vi "Hardware - NI 9755-1 (NOx) Host.vi"() -> ()   [LabVIEW 2015, in "ECS-Host.lvlib"]
uses:
  ECS-Host.lvlib
panel:
  out "RxIDActual":u32 format="%.0x"
  out "FPGAInterfaceError":bool
  in  "Sensor2RxID":u32 format="%.0x"
  out "Sensor2HeaterModeStatus":T1(ring)
  out "Sensor2O2CircuitStatus":enum32{"OPEN WIRE", "SHORT CIRCUIT", "NO ERROR"}(ring)
  out "Sensor2NOxCircuitStatus":enum32{"OPEN WIRE", "SHORT CIRCUIT", "NO ERROR"}(ring)
  out "Sensor2HeaterCircuitStatus":enum32{"OPEN WIRE", "SHORT CIRCUIT", "NO ERROR"}(ring)
  out "Sensor2O2SignalStatus":T2(ring)
  out "Sensor2NOxSignalStatus":T2(ring)
  out "Sensor2TemperatureStatus":T3(ring)
  out "Sensor2O2":sgl caption="[%]"
  out "Sensor2NOx":i32 caption="[ppm]"
  out "Sensor2SupplyStatus":T4(ring)
  in  "Sensor2_E":bool
  out "Sensor2Present":bool
  in  "TxID":u32 format="%.0x"
  in  "Sensor1RxID":u32 format="%.0x"
  out "Sensor1HeaterModeStatus":T1(ring)
  out "Sensor1O2CircuitStatus":enum32{"OPEN WIRE", "SHORT CIRCUIT", "NO ERROR"}(ring)
  out "Sensor1NOxCircuitStatus":enum32{"OPEN WIRE", "SHORT CIRCUIT", "NO ERROR"}(ring)
  out "Sensor1HeaterCircuitStatus":enum32{"OPEN WIRE", "SHORT CIRCUIT", "NO ERROR"}(ring)
  out "Sensor1O2SignalStatus":T2(ring)
  out "Sensor1NOxSignalStatus":T2(ring)
  out "Sensor1TemperatureStatus":T3(ring)
  out "Sensor1O2":sgl caption="[%]"
  out "Sensor1NOx":i32 caption="[ppm]"
  out "Sensor1SupplyStatus":T4(ring)
  in  "Sensor1_E":bool
  out "Sensor1Present":bool
  in  "CAN0_Restart":bool
  # "NOx1"
  # "NOx2"
  # "Rx ID"
  # "Rx ID"
  # "Supply"
  # "Supply"
  # "Temperature"
  # "Temperature"
  # "NOx Signal"
  # "NOx Signal"
  # "O2 Signal"
  # "O2 Signal"
  # "Heater Mode"
  # "Heater Mode"
  # "Heater Circuit"
  # "Heater Circuit"
  # "NOx Circuit"
  # "NOx Circuit"
  # "O2 Circuit"
  # "O2 Circuit"
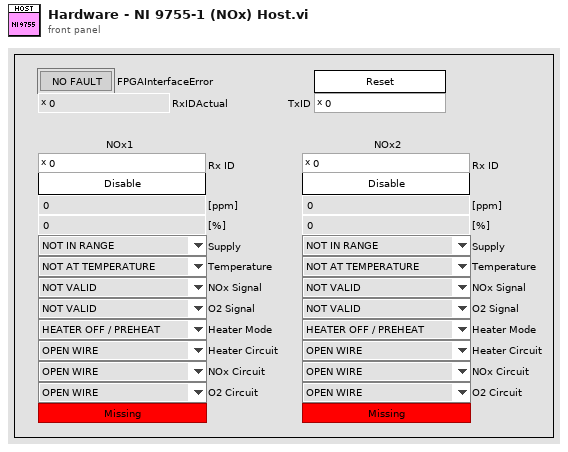
[diagram p1: front panel]
types:
  T1 = enum32{"HEATER OFF / PREHEAT", "HEATER SLOPE 1 OR 2", "HEATER SLOPE 3 OR 4", "AUTO MODE"}
  T2 = enum32{"NOT VALID", "VALID", "ERROR", "NOT AVAILABLE"}
  T3 = enum32{"NOT AT TEMPERATURE", "AT TEMPERATURE", "ERROR", "NOT AVAILABLE"}
  T4 = enum32{"NOT IN RANGE", "SUPPLY IN RANGE", "ERROR", "NOT AVAILABLE"}
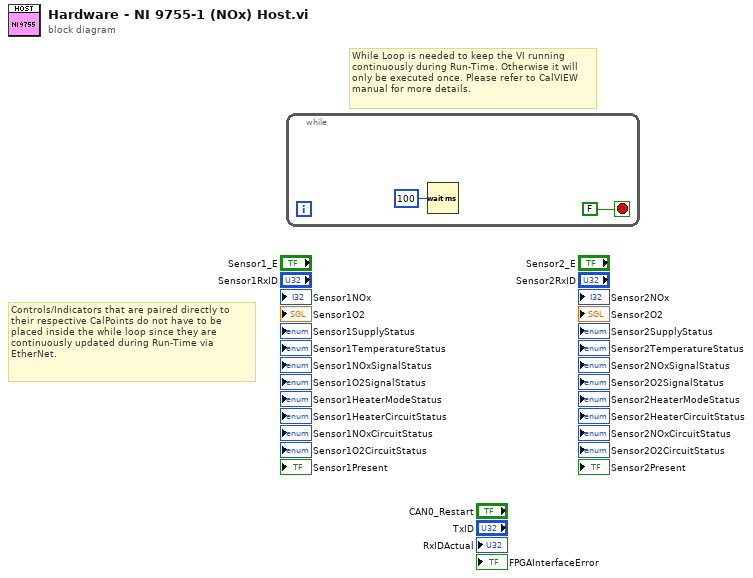
[diagram p0: block diagram]
diagram:
  # "While Loop is needed to keep the VI running\ncontinuously during Run-Time. Otherwise it will only be executed once. Please refer to CalVIEW manual for more details."
  # "Controls/Indicators that are paired directly to their respective CalPoints do not have to be placed inside the while loop since they are continuously updated during Run-Time via EtherNet."
  n1 = while {
    stop <- FALSE stop-if-true
    n2 = Wait (ms)(milliseconds to wait=u32 100) -> ()  [unwired: 1 out]
  }
